vi "DllDriver.vi"() -> ()   [LabVIEW 2010]
panel:
  in  "arg1":i32
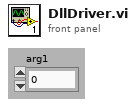
[diagram p1: front panel]
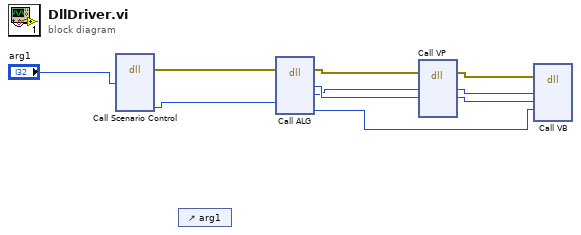
[diagram p0: block diagram]
diagram:
  n1 = dll-call lib="?" fn="Call Scenario Control"("arg1"="arg1") -> (error out=w10:errorcluster, "arg4"=w2:i32)  [unwired: 10 in, 1 out]
  n2 = control-ref of="arg1"() -> ()  [unwired: 1 out]
  n3 = dll-call lib="?" fn="Call ALG"(error in=w10, "arg3"=w2) -> (error out=w9:errorcluster, "arg1"=w7:i32, "arg2"=w6:i32, "arg4"=w3:i32)  [unwired: 7 in, 1 out]
  n4 = dll-call lib="?" fn="Call VP"(error in=w9, "arg1"=w6, "arg2"=w7) -> (error out=w8:errorcluster, "arg1"=w5:i32, "arg2"=w4:i32)  [unwired: 7 in, 1 out]
  n5 = dll-call lib="?" fn="Call VB"(error in=w8, "arg1"=w5, "arg2"=w4, "arg3"=w3) -> ()  [unwired: 8 in, 2 out]
